vi "setUp.vi"(8 "error in":errorcluster, 11 "reference in":refnum<class "Examples.lvclass">) -> (0 "error out":errorcluster, 3 "reference out":refnum<class "Examples.lvclass">)   [LabVIEW 2020, in "Examples.lvclass"]
doc: "setUp runs prior to the test method during test execution. Use this method to initialize any object data required by your tests."
uses:
  Examples.lvclass
  Examples.lvclass/Examples.ctl
  <vilib>/addons/_JKI Toolkits/VI Tester/TestCase.llb/TestCase.lvclass
  <userlib>/_OpenG.lib/appcontrol/appcontrol.llb/openg_application_control.lvlib
  <vilib>/NI/VeriStand Custom Device Testing Tools/VeriStandTestUtilities/VeriStandTestUtilities.lvlib
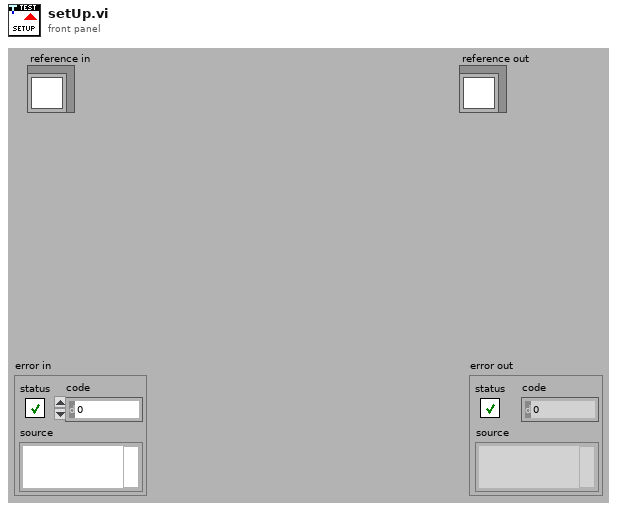
[diagram p1: front panel]
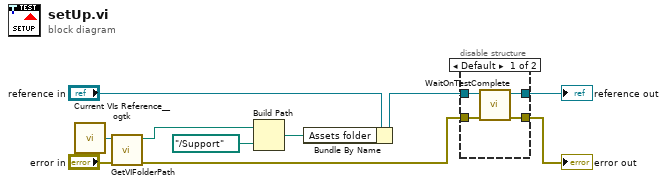
[diagram p0: block diagram]
diagram:
  n1 = call <userlib>:"Current VIs Reference__ogtk.vi"() -> ("Current VI's reference"=w8:refnum<vi>)  [unwired: 5 in]
  n2 = call <vilib>:"GetVIFolderPath.vi"("error in (no error)"="error in", "VI Reference in"=w8) -> ("error out"=w4:errorcluster, "VI Folder Path out"=w7:path)  [unwired: 8 in]
  n3 = Build Path(base path=w7, name or relative path=path "../Support" ("Absolute or Relative Path")) -> (appended path=w5:path)
  n4 = Bundle By Name(cluster="reference in", "Assets folder"=w5) -> (w1:refnum<class "Examples.lvclass">)
  n5 = disable-structure shown="Default" {
    disable-tunnel: w4 -> [w14 w15]
    disable-tunnel: [w13 w15] -> w10
    disable-tunnel: [w12 w16] -> w9
    disable-tunnel: w1 -> [w11 w16]
    frame condition #0 (active) {
      n6 = call <vilib>:"WaitOnTestComplete.vi"("error in (no error)"=w14, "TestCase in"=w11) -> ("error out"=w13:errorcluster, "TestCase out"=w12:refnum<class "Examples.lvclass">)  [unwired: 8 in]
    }
    frame condition #1 {
    }
  }
  "error out" <- w10
  "reference out" <- w9
